vi "EPA_Tabelle zusammenbauen.vi"(8 "error in (no error)":errorcluster caption="Fehler (Eingang, kein Fehler)", 11 "Eingabetabelle":T1) -> (0 "error out":errorcluster caption="Fehler (Ausgang)", 1 "XY-Graph":cluster{dbl[], dbl[]}[](array[cluster]), 3 "EPA Ausgabetabelle":string[][](table))   [LabVIEW 2020, in "Linearisierung v2.lvlib"]
uses:
  Linearisierung v2.lvlib
  Eingabetabelle.ctl
  Aktion Lin Daten aufarbeiten.ctl
panel:
  # "Tabelle:\n0.....Sollwert\n1.....Istwert\n2.....Rohwert\n3.....linearisiert\n4.....abs.Fehler ppm\n5.....Fehler in %\n6.....Deviation\n7.....Temp.Messzelle\n8.....Druck Messzelle\n9.....abs.Fehler ppm linearisiert\n10....Fehler in % linearisiert\n11....abs.Fehler ppm EPA\n12....Fehler in % EPA\n13....abs.Fehler ppm Rohwert\n14....Fehler in % Rohwert"
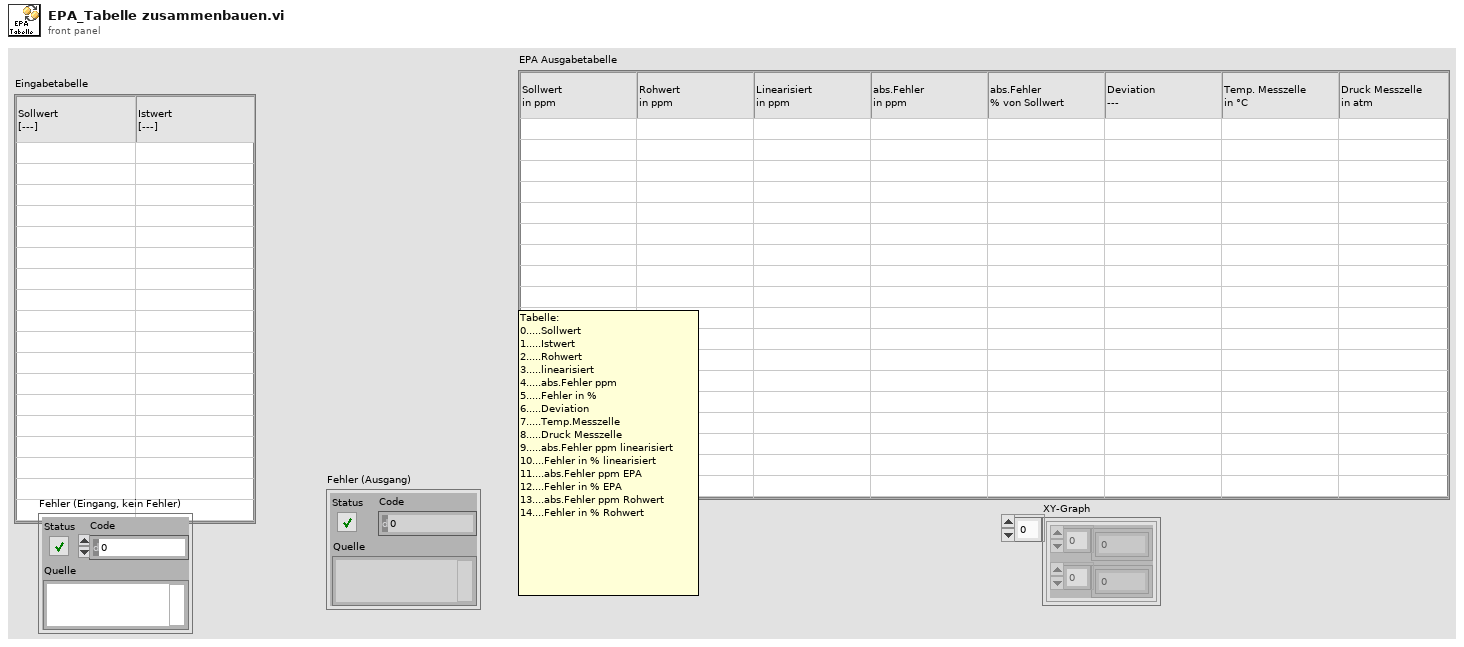
[diagram p1: front panel]
types:
  T1 = typedef "Linearisierung v2.lvlib/Eingabetabelle.ctl" = string[][]
  T2 = typedef "Linearisierung v2.lvlib/Aktion Lin Daten aufarbeiten.ctl" = enum16{"lesen", "Protkolldaten", "speichern", "laden", "EPA auswerten", "Tabelle schreiben", "Lin auswerten", "Tab init", "Stufentabelle", "EPA aktiviert", "Nachbehandlung laden", "Tabelle löschen", "Istwerte löschen", "Zeile löschen", "Zeile einfügen", "LIN aktiviert", "LIN/EPA aktiv laden", "EGAK Tab", "LIN übernehmen", "Tab init ohne Stufen"}
  T3 = typedef "Linearisierung v2.lvlib/Lin-Polynom Daten.ctl" = cluster{"Messgerät":string, "Kalibrator (Gasteiler)":string, "Bearbeiter/in":string, "Komponente":string, "Zeitstempel":timestamp, "F_max gefordert (%)":sgl, "F_max in %":sgl, "F_max in ppm":sgl, "Vorschlag Ordnung":i32, "Polynom OK":bool, "Polynomkoeff.":dbl[], "Prüfgas Konzentration":dbl, "Pfad EPA":string, "Pfad_LIN":string, "Gasnummer:":u8, "Komponentenauswahl":T4, "Verdünnungsgas":T6, "Zeitdauer Stufe":T7, "Anzahl Stufen":T7, "F_max in % EPA":sgl, "F_max in ppm EPA":sgl, "F_max in % LIN":sgl, "F_max in ppm LIN":sgl, "Punkte umkehren":bool, "EPA Optionsfeld":T8, "Autolin Hovacal":T9, "Spanfactors":sgl[], "Kalibrierauswahl":T10, "Conditions:":T11, "Gasflaschen Nr.:":string, "Bottle Accuracy":dbl, "Konfig Gasflasche":T12, "Gasflasche":T13, "HovaCAL Flow AutoLin":T14, "MFC Output":T15, "Gas Ablaufdatum":timestamp, "Lin Modus":T16, "zusätzliche Zeitdauer Erster Punkt":sgl, "Offsets":sgl[]}
  T4 = typedef "Linearisierung v2.lvlib/KomponentenArray.ctl" = cluster{"Komponente:":T5, "Konzentration":dbl}[]
  T5 = typedef "Auswahlfeld.ctl" = u16
  T6 = typedef "Linearisierung v2.lvlib/Gasteiler.lvlib/Prüfgas in.ctl" = u16
  T7 = typedef "Zahlen-Eingabefeld.ctl" = sgl
  T8 = typedef "Linearisierung v2.lvlib/EPA Optionsfeld.ctl" = enum32{"Istwert", "Rohwert", "Linearisierter Wert"}
  T9 = typedef "Linearisierung v2.lvlib/Gasteiler.lvlib/HovaCal.lvlib/AutoLin Hovacal.ctl" = enum32{"Keine Auswahl", "Optionsauswahl 1", "Optionsauswahl 2"}
  T10 = typedef "Linearisierung v2.lvlib/Kalibrieroption.ctl" = u16
  T11 = typedef "Linearisierung v2.lvlib/Linearity verification 1065-307.lvlib/Condition.ctl" = u16
  T12 = typedef "System Einstellungen V2.lvlib/Konfig Gasflasche.ctl" = bool
  T13 = typedef "System Einstellungen V2.lvlib/Gasflasche Auswahl.ctl" = u16
  T14 = typedef "Linearisierung v2.lvlib/Gasteiler.lvlib/HovaCAL_Interface.lvlib/Controls.lvlib/Flow Einstellung.ctl" = cluster{"HovaCAL Flow Input Cluster":dbl}
  T15 = typedef "Linearisierung v2.lvlib/Gasteiler.lvlib/HovaCAL_Interface.lvlib/Controls.lvlib/Pump state.ctl" = cluster{"Run":bool}
  T16 = typedef "CalGas Aufschaltung.lvlib/Lin Modus.ctl" = u16
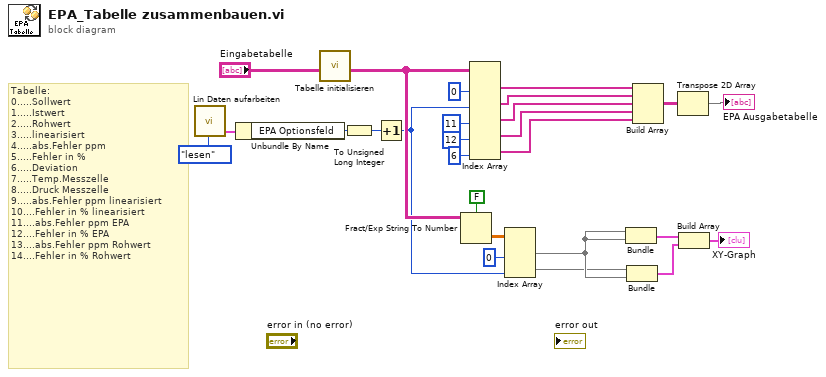
[diagram p0: block diagram]
diagram:
  # "Tabelle:\n0.....Sollwert\n1.....Istwert\n2.....Rohwert\n3.....linearisiert\n4.....abs.Fehler ppm\n5.....Fehler in %\n6.....Deviation\n7.....Temp.Messzelle\n8.....Druck Messzelle\n9.....abs.Fehler ppm linearisiert\n10....Fehler in % linearisiert\n11....abs.Fehler ppm EPA\n12....Fehler in % EPA\n13....abs.Fehler ppm Rohwert\n14....Fehler in % Rohwert"
  n1 = call "Lin Daten aufarbeiten.vi"("Aktionen"=Aktion_Lin_Daten_aufarbeiten."lesen") -> ("Lin-Polynom"=w5:T3)  [unwired: 16 in, 10 out]
  n2 = Unbundle By Name(w5) -> ("EPA Optionsfeld"=w4:T8)
  n3 = call "Tabelle initialisieren.vi"("Neue Tabelle"="Eingabetabelle") -> ("Tabelle"=w7:string[][])  [unwired: 10 in]
  n4 = To Unsigned Long Integer(number=w4) -> (unsigned 32bit integer=w3:u32)
  n5 = Increment(x=w3) -> (x+1=w2:u32)
  n6 = Fract/Exp String To Number(use system decimal point (T)=FALSE ("Systemdezimalzeichen verwenden (T)"), string=w7) -> (number=w13:dbl[][])  [unwired: 2 in, 1 out]
  n7 = Index Array(array=w7, index (col) #1=0 ("Deaktivierter Index (Spalte)"), index (col) #2=w2, index (col) #3=11 ("Index (Spalte)"), index (col) #4=12 ("Index (Spalte)"), index (col) #5=6 ("Index (Spalte)")) -> (element #1=w16:string[], element #2=w17:string[], element #3=w24:string[], element #4=w21:string[], element #5=w20:string[])  [unwired: 5 in]
  n8 = Index Array(array=w13, index (col) #1=0 ("Deaktivierter Index (Spalte)"), index (col) #2=w2) -> (element #1=w11:dbl[], element #2=w10:dbl[])  [unwired: 2 in]
  n9 = Bundle(w11, w11) -> (w15:cluster{dbl[], dbl[]})  [unwired: 1 in]
  n10 = Bundle(w10, w11) -> (w14:cluster{dbl[], dbl[]})  [unwired: 1 in]
  n11 = Build Array(w16, w17, w24, w21, w20) -> (w19:string[][])
  n12 = Transpose 2D Array(2D array=w19) -> (transposed array=→"EPA Ausgabetabelle":string[][])
  n13 = Build Array(w15, w14) -> (→"XY-Graph":cluster{dbl[], dbl[]}[])
